vi "Unregister Sessions Wrapper.vi"(8 "error in":errorcluster, 11 "request data":T2) -> (0 "error out":errorcluster, 3 "response data":T1)   [LabVIEW 2020, in "Measurement Plugin Session Management V1.lvlib" / "Session Reservation.lvclass"]
uses:
  Session Reservation.lvclass
  Measurement Plugin Session Management Client/RPC Messages/ni_measurementlink_sessionmanagement_v1_UnregisterSessionsRequest.ctl
  Measurement Plugin Session Management Client/RPC Messages/ni_measurementlink_sessionmanagement_v1_SessionInformation.ctl
  Measurement Plugin Session Management Client/RPC Messages/nidevice_grpc_Session.ctl
  Measurement Plugin Session Management Client/RPC Messages/ni_measurementlink_sessionmanagement_v1_ChannelMapping.ctl
  Measurement Plugin Session Management Client/RPC Messages/ni_measurementlink_sessionmanagement_v1_UnregisterSessionsResponse.ctl
  Measurement Plugin Discovery V1/TypeDefs/gRPC Client Cache FGV Action.ctl
  Measurement Plugin Discovery V1/Measurement Plugin Discovery V1.lvlib
  Measurement Plugin Session Management Client/Measurement Plugin Session Management Client.lvlib
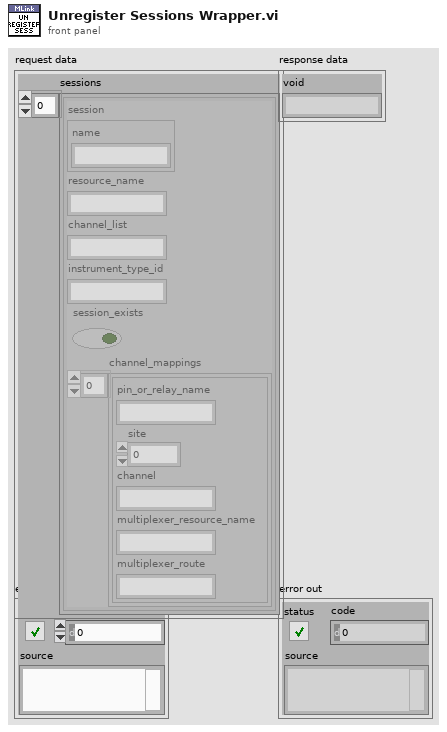
[diagram p1: front panel]
types:
  T1 = typedef "Measurement Plugin Session Management Client.lvlib/ni_measurementlink_sessionmanagement_v1_UnregisterSessionsResponse.ctl" = cluster{"void":string}
  T2 = typedef "Measurement Plugin Session Management Client.lvlib/ni_measurementlink_sessionmanagement_v1_UnregisterSessionsRequest.ctl" = cluster{"sessions":T3[]}
  T3 = typedef "Measurement Plugin Session Management Client.lvlib/ni_measurementlink_sessionmanagement_v1_SessionInformation.ctl" = cluster{"session":T4, "resource_name":string, "channel_list":string, "instrument_type_id":string, "session_exists":bool, "channel_mappings":T5[]}
  T4 = typedef "Measurement Plugin Session Management Client.lvlib/nidevice_grpc_Session.ctl" = cluster{"name":string}
  T5 = typedef "Measurement Plugin Session Management Client.lvlib/ni_measurementlink_sessionmanagement_v1_ChannelMapping.ctl" = cluster{"pin_or_relay_name":string, "site":i32, "channel":string, "multiplexer_resource_name":string, "multiplexer_route":string}
  T6 = typedef "Measurement Plugin Discovery V1.lvlib/gRPC Client Cache FGV Action.ctl" = enum16{"Get Client", "Recreate Client", "Destroy Client", "Update ClusterId"}
  T7 = typedef "grpc-lvsupport-release.lvlib/grpcId.ctl" = u64
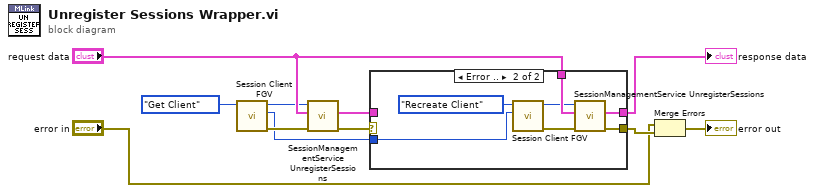
[diagram p0: block diagram]
diagram:
  n1 = call "Session Client FGV.vi"("action"=gRPC_Client_Cache_FGV_Action."Get Client") -> ("error out"=w8:errorcluster, "unique id out"=w3:u64, "grpc client id"=w4:T7)  [unwired: 8 in]
  n2 = call "SessionManagementService UnregisterSessions.vi"("error in"=w8, "Request Data"="request data", "gRPC ID"=w4) -> ("error out"=w7:errorcluster, "Response Data"=w5:T1)  [unwired: 6 in, 1 out]
  n3 = case shown="Error .." w7 {
    selector: w7 -> [w13 _]
    tunnel: [w13 w19] -> w11
    tunnel: [w12 w18] -> w9
    tunnel: w5 -> [w12 _]
    tunnel: "request data" -> [_ w17]
    tunnel: w3 -> [_ w14]
    frame No Error {
    }
    frame Error {
      n4 = call "Session Client FGV.vi"("unique id in"=w14, "action"=gRPC_Client_Cache_FGV_Action."Recreate Client") -> ("error out"=w20:errorcluster, "grpc client id"=w16:T7)  [unwired: 7 in, 1 out]
      n5 = call "SessionManagementService UnregisterSessions.vi"("error in"=w20, "Request Data"=w17, "gRPC ID"=w16) -> ("error out"=w19:errorcluster, "Response Data"=w18:T1)  [unwired: 6 in, 1 out]
    }
  }
  "response data" <- w9
  n6 = Merge Errors("error in", w11) -> (→"error out":errorcluster)
